vi "Demo Combo Box.vi"(8 "error in (no error)":errorcluster) -> (0 "error out":errorcluster)   [LabVIEW 2011]
uses:
  VIremote.llb/VIremoteEvent.ctl
  VIremote.llb/VIremoteFunction.ctl
panel:
  in  "Combo Box 3":string(combo)="First item" caption="Combo Box Grouped"
  in  "Combo Box 2":string(combo)="First item" caption="Combo Box"
  in  "Combo Box":string(combo)="First item" caption="Allow undefined strings"
  in  "VIremoteEvent":T1=enum."Connection Closed"
  # "Tap anywhere on the combo box above to display an iOS-picker to change its value. \n\nThe combo box below has \"Allow undefined strings\" checked and if you tap the string it can be edited. If you tap the arrow the picker will be displayed."
  # "You can customize the style and other properites of the popup  in the description (default is picker). This one has Style=Grouped. See the Ring and Enum demo for mor examples."
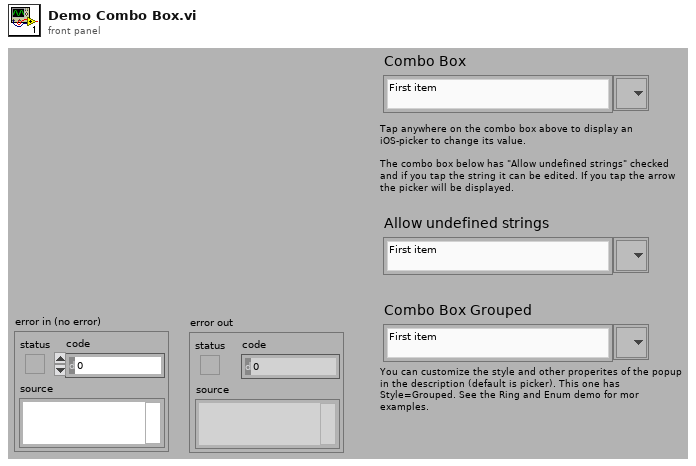
[diagram p1: front panel]
types:
  T1 = typedef "VIremoteEvent.ctl" = enum16{"No Event", "Connection Closed", "Navigate Back", "Enter Background", "Enter Foreground", "Portrait", "Portrait Upside Down", "Landscape Left", "Landscape Right"}
  T2 = typedef "VIremoteFunction.ctl" = enum16{"Do nothing", "Stop controller", "Close this connection", "Show info panel", "Set VI to control", "Set Accelerometer freq (Hz)", "Show Alert message", "Start Sound Input", "Stop Sound Input", "Set Volume (0-100)", "Set sound output Speaker", "Set sound output Receiver", "Play Sound", "Repeat Sound", "Stop Sound", "Pause Sound", "Resume Sound", "Set panel width of caller (320 or 480)", "Set Panel Size to Portrait", "Set Panel Size to Landscape", "Set Panel Size as Current Orientation", "Allow all UI Orientations", "Send user notification", "Disable Scrolling", "Normal Scrolling", "Page Scrolling", "Set Scroll Offset", "Page Indicator Position"}
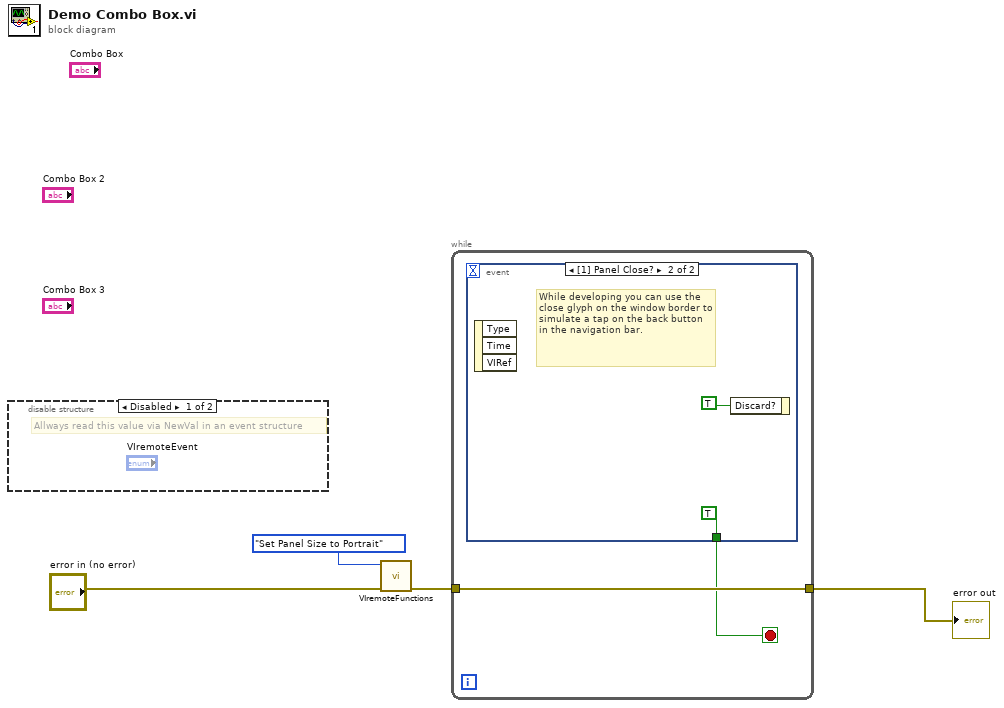
[diagram p0: block diagram]
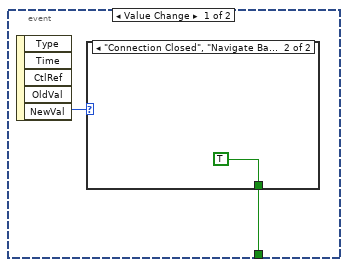
[diagram p3: hidden frame]
diagram:
  n1 = disable-structure shown="Disabled" {
    frame Disabled {
      # "Allways read this value via NewVal in an event structure"
    }
    frame Enabled {
    }
  }
  n2 = call "VIremoteFunctions.vi"("error in (no error)"="error in (no error)", "Function"=VIremoteFunction."Set Panel Size to Portrait") -> ("error out"=w3:errorcluster)  [unwired: 4 in, 5 out]
  n3 = while {
    tunnel: [w6] -> w1
    tunnel: w3 -> [w6]
    stop <- w5 stop-if-true
    n4 = event shown="[1] Panel Close?" {
      selector: _ -> [_ _]
      dyn-events: _ -> [_ _]
      timeout: _ -> [_ _]
      tunnel: [w7 TRUE ("Discard?")] -> w5
      event Value Change {
        n5 = event-data() -> ("NewVal"=w8:T1)  [unwired: 5 out]
        n6 = case shown="\"Connection Closed\", \"Navigate Back\"" w8 {
          tunnel: [_ TRUE] -> w7
          frame "No Event", Default {
          }
          frame "Connection Closed", "Navigate Back" {
          }
        }
      }
      event Panel Close? {
        # "While developing you can use the close glyph on the window border to simulate a tap on the back button in the navigation bar."
        n7 = event-data() -> ()  [unwired: 4 out]
        n8 = event-data("Discard?"=TRUE) -> ()  [unwired: 1 in, 1 out]
      }
    }
  }
  "error out" <- w1
